vi "Write Signal Amplitude to State.vi"(8 "error in (no error)":errorcluster, 10 "amplitude":dbl, 11 "SV Signal in":refnum<class "SV Signal.lvclass">) -> (0 "error out":errorcluster, 3 "SV Signal out":refnum<class "SV Signal.lvclass">)   [LabVIEW 2017, in "SV Signal.lvclass"]
uses:
  <vilib>/addons/_NISVFA/_Generation/Signal Generation/SV Signal/SV Signal.lvclass
  <vilib>/addons/_NISVFA/_Generation/Signal Generation/SV Signal/sv_Signal State Attribute.ctl
  <vilib>/addons/_NISVFA/_Generation/Signal Generation/SV Signal/SV Signal.lvclass/SV Signal.ctl
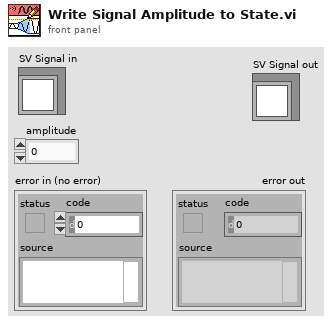
[diagram p1: front panel]
types:
  T1 = typedef "SV Signal.lvclass/sv_Signal State Attribute.ctl" = string
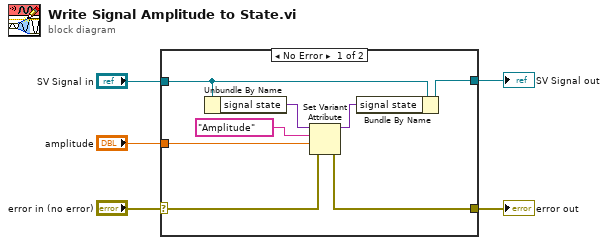
[diagram p0: block diagram]
diagram:
  n1 = case shown="No Error" "error in (no error)" {
    selector: "error in (no error)" -> [w6 w14]
    tunnel: "amplitude" -> [w13 _]
    tunnel: "SV Signal in" -> [w9 w15]
    tunnel: [w8 w15] -> w3
    tunnel: [w7 w14] -> w2
    frame No Error {
      n2 = Unbundle By Name(w9) -> ("signal state"=w10:variant)
      n3 = Set Variant Attribute(Variant=w10, name=T1 "Amplitude", value=w13, error in=w6) -> (Variant out=w11:variant, error out=w7:errorcluster)  [unwired: 1 out]
      n4 = Bundle By Name(cluster=w9, "signal state"=w11) -> (w8:refnum<class "SV Signal.lvclass">)
    }
    frame Error {
    }
  }
  "SV Signal out" <- w3
  "error out" <- w2
